vi "Average Measure (More).vi"(0 "VISA resource name":refnum<visa-resource-name>, 5 "Channel (1: Channel 1)":i32(ring)=1 items=["Channel 1"=1, "Channel 2"=2, "Channel 3"=3, "Channel 4"=4, "Function 1"=5, "Function 2"=6, "Function 3"=7, "Function 4"=8, "Memory 1"=9, "Memory 2"=10, "Memory 3"=11, "Memory 4"=12], 7 "Measurement Function (0: Rise Time)":i32(ring) items=["Rise Time", "Fall Time", "Frequency", "Period", "Voltage RMS(AC)", "Voltage RMS(DC)", "Voltage RMS (AC,cycle)", "Voltage RMS (DC,cycle)", "Voltage Max", "Voltage Min", "Voltage Middle", "Voltage Vpp", "Voltage High", "Voltage Low", "Voltage Average", "Voltage Average (cycle)", "Width Negative", "Width Positive", "Duty Cycle Positive", "Amplitude", "Overshoot", "Preshoot", "Voltage Base", "Voltage Upper", "Time Max", "Time Min", "Color Grade Crossing", "Color Grade Eye Width", "Color Grade Eye Height", "Color Grade Eye Q-Factory", "Color Grade Eye Duty Cycle Distortion(Percent)", "Color Grade Eye Duty Cycle Distortion(Time)", "Color Grade Eye Jitter(PP)", "Color Grade Eye Width(RMS)", "Cycle-cycle Duty Jitter(Rising)", "Cycle-cycle Duty Jitter(Falling)", "Cycle-cycle Jitter(Rising)", "Cycle-cycle Jitter(Falling)", "Cycle-cycle - Width", "Cycle-cycle + Width", "Date Rate", "Unit Interval", "FFT Delta Frequency", "FFT Delta Magnitude", "FFT Frequency", "FFT Magnitude", "Slew Rate", "Area (Entire Display)", "Area(Single Cycle)", "Duty Cycle (Rising)", "Duty Cycle (Falling)"], 9 "Maximum Time (10000ms)":u32=10000, 11 "error in (no error)":errorcluster, 12 "Averages":u32=32, 13 "Max Errors":u32=40) -> (4 "VISA resource name out":refnum<visa-resource-name>, 6 "Measure Average":dbl caption="Measurement", 8 "Measure Error":dbl caption="Measurement", 15 "error out":errorcluster)   [LabVIEW 2009]
uses:
  <instrlib>/Agilent 8000 Series/Public/Data/Read Measurement (More).vi
  <instrlib>/Agilent 8000 Series/Agilent 8000 Series.lvlib
  <vilib>/Analysis/NI_AALBase.lvlib
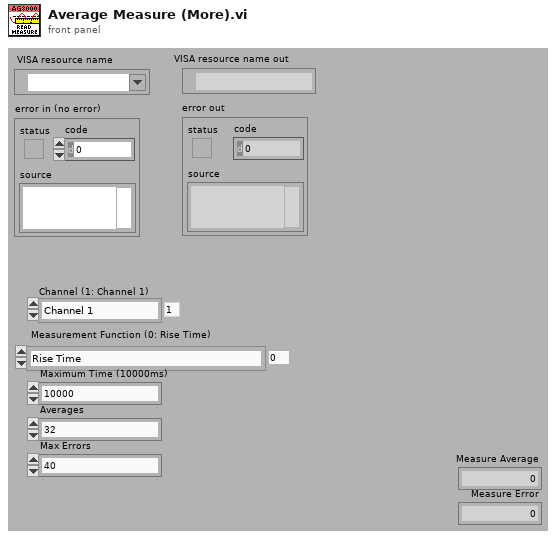
[diagram p1: front panel]
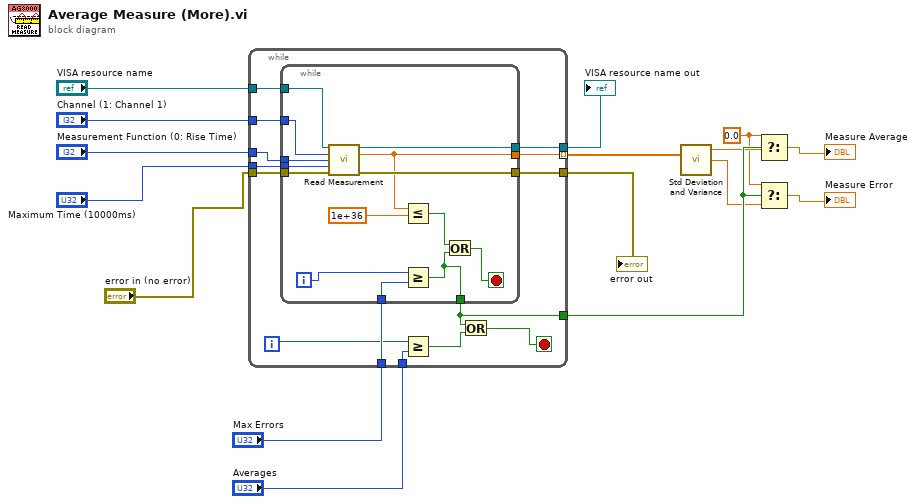
[diagram p0: block diagram]
diagram:
  w3 = 0.0 ("t")
  n1 = while {
    tunnel: "VISA resource name" -> [w30]
    tunnel: "Channel (1: Channel 1)" -> [w17]
    tunnel: "Measurement Function (0: Rise Time)" -> [w29]
    tunnel: "Maximum Time (10000ms)" -> [w28]
    tunnel: "error in (no error)" -> [w27]
    tunnel: [w26] -> w11
    tunnel: [w25] -> w7 mode=indexing
    tunnel: [w24] -> w10
    tunnel: "Max Errors" -> [w23]
    tunnel: "Averages" -> [w21]
    tunnel: [w18] -> w6
    i -> [w22]
    stop <- w19 stop-if-true
    n2 = while {
      tunnel: w30 -> [w44]
      tunnel: w29 -> [w43]
      tunnel: w28 -> [w42]
      tunnel: w27 -> [w41]
      tunnel: [w40] -> w26
      tunnel: [w38] -> w25
      tunnel: [w39] -> w24
      tunnel: w23 -> [w34]
      tunnel: [w32] -> w18
      tunnel: w17 -> [w31]
      i -> [w35]
      stop <- w33 stop-if-true
      n3 = call-poly <instrlib>:"Read Measurement.vi"("VISA resource name"=w44, "Channel (1: Channel 1)"=w31, "Measurement Function (0: Rise Time)"=w43, "Maximum Time (10000ms)"=w42, "error in (no error)"=w41) -> ("VISA resource name out"=w39:refnum<visa-resource-name>, "Measurement"=w38:dbl, "error out"=w40:errorcluster)  [unwired: 8 in]
      n4 = Less Or Equal?(x=w38, y=1e+36) -> (x <= y?=w37:bool)
      n5 = Greater Or Equal?(x=w35, y=w34) -> (x >= y?=w32:bool)
      n6 = Or(x=w37, y=w32) -> (x .or. y?=w33:bool)
    }
    n7 = Greater Or Equal?(x=w22, y=w21) -> (x >= y?=w20:bool)
    n8 = Or(x=w18, y=w20) -> (x .or. y?=w19:bool)
  }
  "error out" <- w11
  "VISA resource name out" <- w10
  n9 = call <vilib>:"Std Deviation and Variance.vi"("X"=w7) -> ("mean"=w4:dbl, "standard deviation"=w5:dbl)  [unwired: 1 in, 1 out]
  n10 = Select(t=w3, s=w6, f=w4) -> (s? t:f=→"Measure Average":dbl)
  n11 = Select(t=w3, s=w6, f=w5) -> (s? t:f=→"Measure Error":dbl)
